vi "Append To Dataset 3D Double.vi"(8 "Number of data points":u64, 9 "data":dbl[][][](array[numeric]), 10 "dataset_id":i32, 11 "error in (no error)":errorcluster) -> (0 "Error code":i32, 3 "error out":errorcluster)   [LabVIEW 2010]
uses:
  Release/HDF5Tools.dll
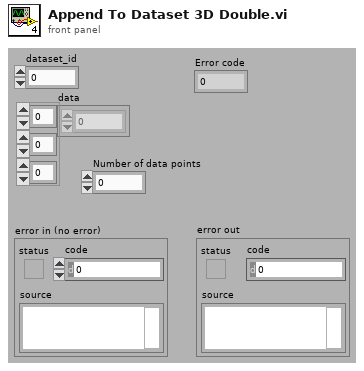
[diagram p1: front panel]
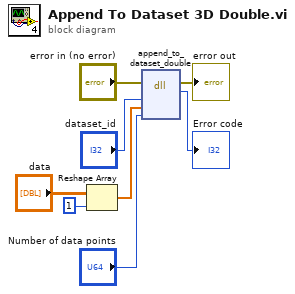
[diagram p0: block diagram]
diagram:
  n1 = Reshape Array("data", 1 ("dimension size")) -> (w1:dbl[])
  n2 = dll-call lib="Z:/users/alex/projects/HDF5Tools/Release/HDF5Tools.dll" fn="append_to_dataset_double"(error in="error in (no error)", "dataset_id"="dataset_id", "data"=w1, "count"="Number of data points") -> (error out=→"error out":errorcluster, "error"=→"Error code":i32)  [unwired: 5 in, 1 out]
